vi "ICA_14_Potluri.vi"   [LabVIEW 2016]
uses:
  <vilib>/NXT/Block Support/NXT_OutputPort.ctl
  <vilib>/NXT/NXTIO Xnodes/NXTIONodeSubVIs/LEGOMoveAllMotorsDistance.vi
  <vilib>/NXT/Dual Mode Library/Waits/Wait_Num.vi
  <vilib>/NXT/NXTIO Xnodes/NXTIONodeSubVIs/NXTMotorRunDistance.vi
  <vilib>/NXT/Dual Mode Library/Sensors/Touch_Pressed.vi
  <vilib>/NXT/Dual Mode Library/Waits/Wait_Num(msec).vi
  <vilib>/NXT/NXTIO Xnodes/NXTIONodeSubVIs/LEGOMoveAllMotors.vi
  <vilib>/NXT/NXTIO Xnodes/NXTIONodeSubVIs/LEGOStopAllMotors.vi
  <vilib>/NXT/Subs/LVHSConnector.ctl
  <vilib>/NXT/NXTIO Xnodes/NXTIOXNode/NXTIO.xnode
  <vilib>/NXT/NXTIO Xnodes/AddressXNode/NXTIOAddress.xnode
  <vilib>/NXT/LegoClasses/BrickReference/BrickReference.lvclass
types:
  T1 = typedef "LVHSConnector.ctl" = refnum<class "BrickReference.lvclass">
  T2 = typedef "NXT_OutputPort.ctl" = u8
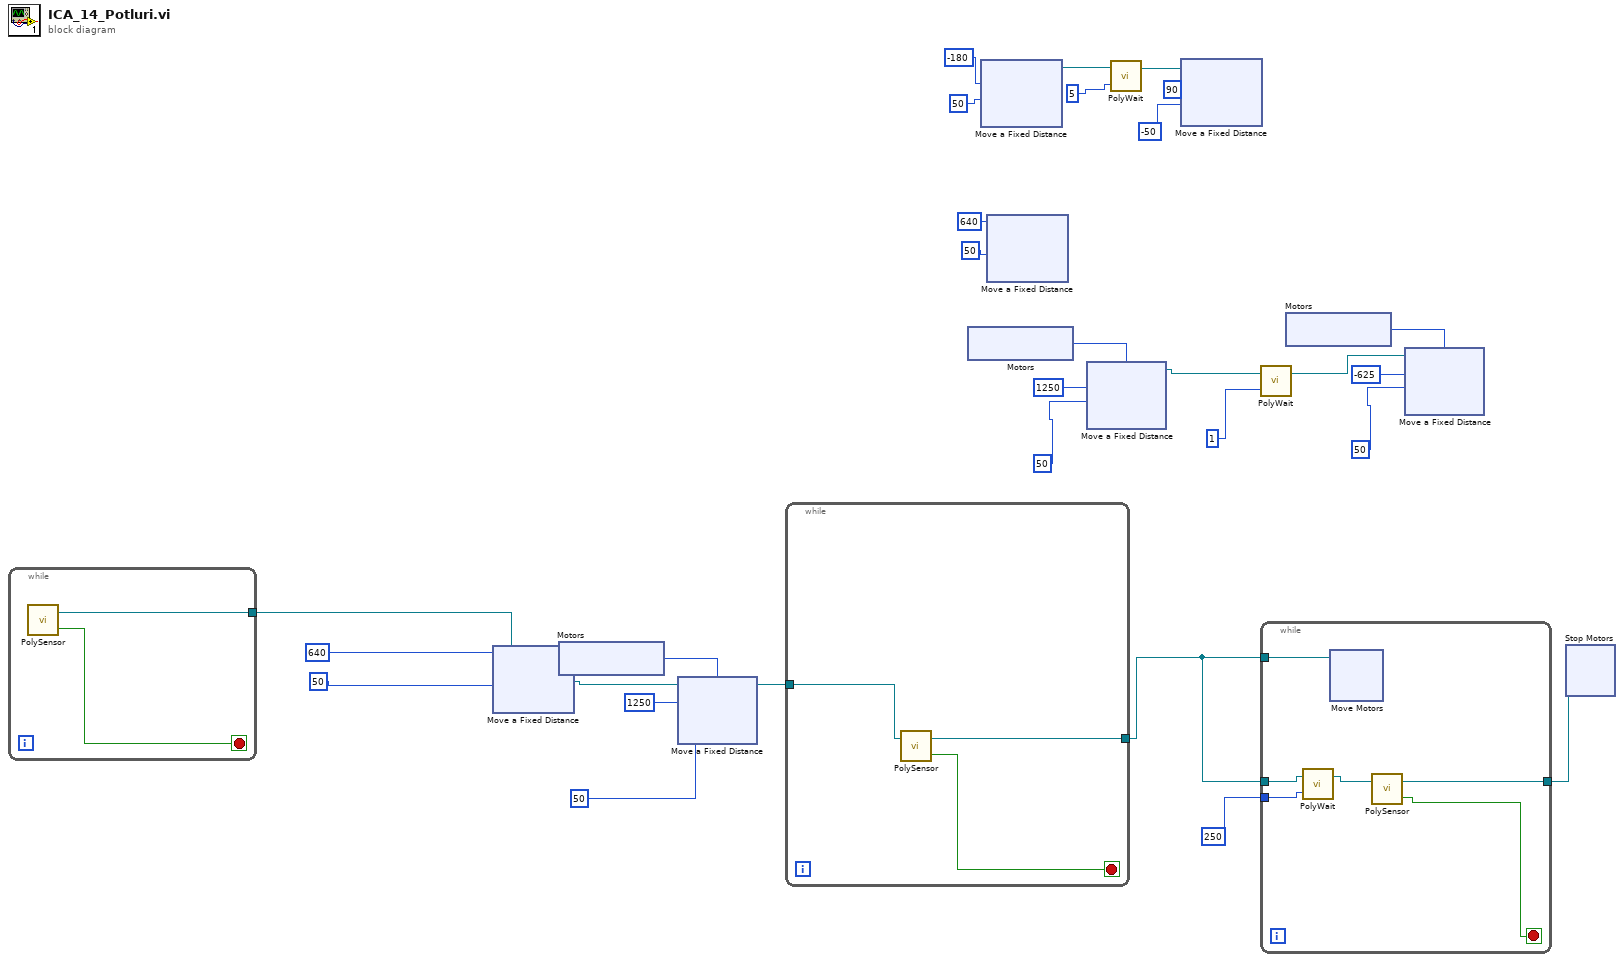
[diagram p0: block diagram]
diagram:
  n1 = while {
    tunnel: [w31] -> w1
    stop <- w30 stop-if-true
    n2 = call-poly <vilib>:"PolySensor.vi"() -> ("Yes / No"=w30:bool, "NXT/EV3"=w31:T1)  [unwired: 3 in]
  }
  n3 = xnode "Move a Fixed Distance"("Speed 1"=50, "Distance 1"=640, "NXT/EV3"=w1) -> ("NXT/EV3"=w7:T1)  [unwired: 1 in]
  n4 = xnode "Motors"() -> ("Motor"=w8:T2)
  n5 = xnode "Move a Fixed Distance"("Speed 1"=50, "Distance 1"=1250, "Motors"=w8, "NXT/EV3"=w7) -> ("NXT/EV3"=w5:T1)
  n6 = while {
    tunnel: [w34] -> w3
    tunnel: w5 -> [w32]
    stop <- w33 stop-if-true
    n7 = call-poly <vilib>:"PolySensor.vi"("NXT/EV3"=w32) -> ("Yes / No"=w33:bool, "NXT/EV3"=w34:T1)  [unwired: 2 in]
  }
  n8 = xnode "Motors"() -> ("Motor"=w18:T2)
  n9 = xnode "Move a Fixed Distance"("Speed 1"=50, "Distance 1"=-180) -> ("NXT/EV3"=w27:T1)  [unwired: 2 in]
  n10 = xnode "Move a Fixed Distance"("Speed 1"=50, "Distance 1"=640) -> ()  [unwired: 2 in, 1 out]
  n11 = xnode "Move a Fixed Distance"("Speed 1"=50, "Distance 1"=1250, "Motors"=w18) -> ("NXT/EV3"=w17:T1)  [unwired: 1 in]
  n12 = call-poly <vilib>:"PolyWait.vi"("Time (1 sec)"=5, "NXT/EV3"=w27) -> ("NXT/EV3"=w25:T1)  [unwired: 2 in]
  n13 = xnode "Move a Fixed Distance"("Speed 1"=-50, "Distance 1"=90, "NXT/EV3"=w25) -> ()  [unwired: 1 in, 1 out]
  n14 = call-poly <vilib>:"PolyWait.vi"("Time (1 sec)"=1, "NXT/EV3"=w17) -> ("NXT/EV3"=w13:T1)  [unwired: 2 in]
  n15 = while {
    tunnel: w3 -> [w40]
    tunnel: [w38] -> w4
    tunnel: w3 -> [w37]
    tunnel: 250 -> [w35]
    stop <- w39 stop-if-true
    n16 = call-poly <vilib>:"PolyWait.vi"("Time (100 msec)"=w35, "NXT/EV3"=w37) -> ("NXT/EV3"=w36:T1)  [unwired: 2 in]
    n17 = xnode "Move Motors"("NXT/EV3"=w40) -> ()  [unwired: 2 in, 1 out]
    n18 = call-poly <vilib>:"PolySensor.vi"("NXT/EV3"=w36) -> ("Yes / No"=w39:bool, "NXT/EV3"=w38:T1)  [unwired: 2 in]
  }
  n19 = xnode "Motors"() -> ("Motor"=w12:T2)
  n20 = xnode "Move a Fixed Distance"("Speed 1"=50, "Distance 1"=-625, "Motors"=w12, "NXT/EV3"=w13) -> ()  [unwired: 1 out]
  n21 = xnode "Stop Motors"("NXT/EV3"=w4) -> ()  [unwired: 1 in, 1 out]
